vi "Write Export Config File.vi"(8 "error in (no error)":errorcluster, 10 "Export Definition File Path":path, 11 "Export in":refnum<class "Export.lvclass">) -> (0 "error out":errorcluster, 3 "Export out":refnum<class "Export.lvclass">)   [LabVIEW 2017, in "CL_G3_VIComponentBuilder.lvlib" / "Export.lvclass"]
uses:
  Export.lvclass
  Export.lvclass/Export.ctl
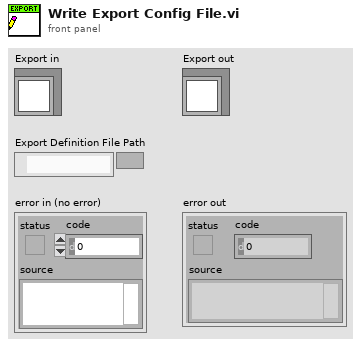
[diagram p1: front panel]
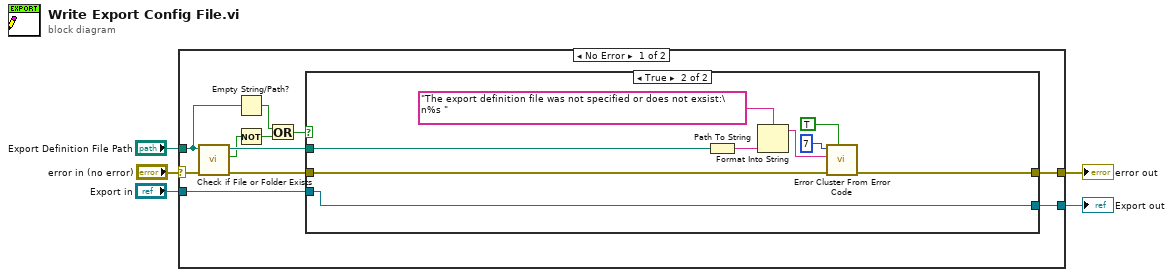
[diagram p0: block diagram]
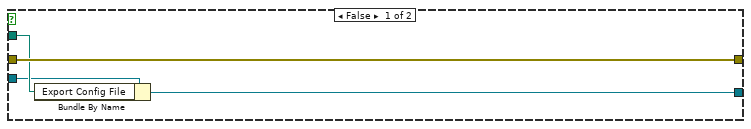
[diagram p2: hidden frame]
diagram:
  n1 = case shown="No Error" "error in (no error)" {
    selector: "error in (no error)" -> [w14 w30]
    tunnel: [w12 w30] -> w4
    tunnel: [w15 w31] -> w2
    tunnel: "Export in" -> [w16 w31]
    tunnel: "Export Definition File Path" -> [w10 _]
    frame No Error {
      n2 = call <vilib>:"Check if File or Folder Exists.vi"("error in (no error)"=w14, "path"=w10) -> ("error out"=w11:errorcluster, "file or folder exists?"=w9:bool, "dup path"=w13:path)  [unwired: 7 in]
      n3 = Empty String/Path?(string/path=w10) -> (empty?=w6:bool)
      n4 = Not(x=w9) -> (.not. x?=w8:bool)
      n5 = Or(x=w6, y=w8) -> (x .or. y?=w7:bool)
      n6 = case shown="True" w7 {
        tunnel: w16 -> [w18 w29]
        tunnel: [w17 w29] -> w15
        tunnel: w13 -> [w19 w28]
        tunnel: [w20 w21] -> w12
        tunnel: w11 -> [w20 w22]
        frame False {
          n7 = Bundle By Name(cluster=w18, "Export Config File"=w19) -> (w17:refnum<class "Export.lvclass">)
        }
        frame True {
          n8 = Path To String(path=w28) -> (string=w27:string)
          n9 = Format Into String(format string="The export definition file was not specified or does not exsist:\n%s ", w27) -> (resulting string=w23:string)  [unwired: 2 in, 1 out]
          n10 = call <vilib>:"Error Cluster From Error Code.vi"("show call chain? (False)"=TRUE, "error in (no error)"=w22, "error message (\"\")"=w23, "error code (0)"=7) -> ("error out"=w21:errorcluster)  [unwired: 5 in]
        }
      }
    }
    frame Error {
    }
  }
  "error out" <- w4
  "Export out" <- w2
